vi "Setup.vi"(8 "error in (no error)":errorcluster, 11 "Test Case In":refnum<class "Animal Test.lvclass">) -> (0 "error out":errorcluster, 3 "Test Case Out":refnum<class "Animal Test.lvclass">)   [LabVIEW 2020, in "Animal Test.lvclass"]
doc: "Setup"
uses:
  Animal Test.lvclass
  Animal Classes/Animal/Animal.lvclass
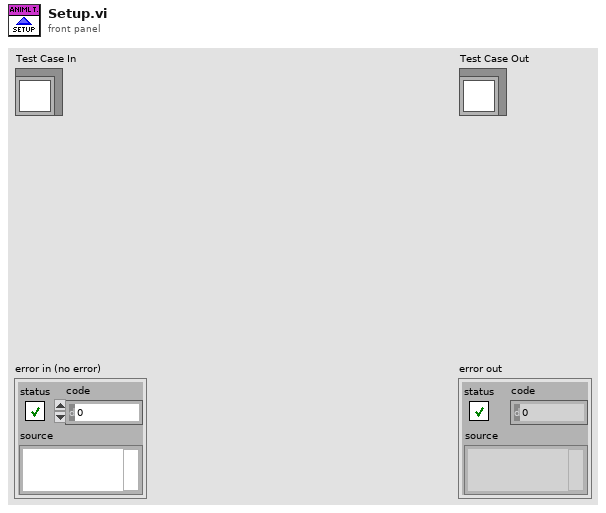
[diagram p1: front panel]
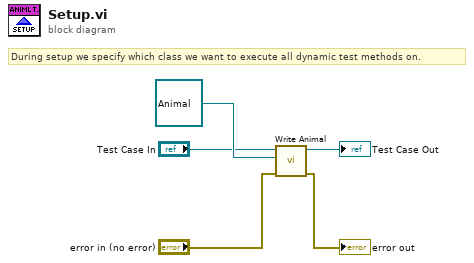
[diagram p0: block diagram]
diagram:
  # "During setup we specify which class we want to execute all dynamic test methods on."
  n1 = call "Write Animal.vi"("error in (no error)"="error in (no error)", "Animal.lvclass"=refnum<class "Animal.lvclass"> refnum, "Animal Test In"="Test Case In") -> ("error out"=→"error out":errorcluster, "Animal Test Out"=→"Test Case Out":refnum<class "Animal Test.lvclass">)  [unwired: 7 in]
